vi "Destroy_ErrorHandler.vi"(8 "error in (no error)":errorcluster, 11 "ErrorHandler in":refnum<class "ErrorHandler.lvclass">) -> (0 "error out":errorcluster, 3 "ErrorHandler out":refnum<class "ErrorHandler.lvclass">)   [LabVIEW 2017, in "ErrorHandler.lvclass"]
doc: "Developed by Kevin Thompson\nkevin@thompsonengineering.net\n\nCopyright 2018\nThompson Engineering, LLC"
uses:
  ErrorHandler.lvclass
  TypeDef/TD GetSet ActionSelect--enum.ctl
  ErrorHandler.lvclass/ErrorHandler.ctl
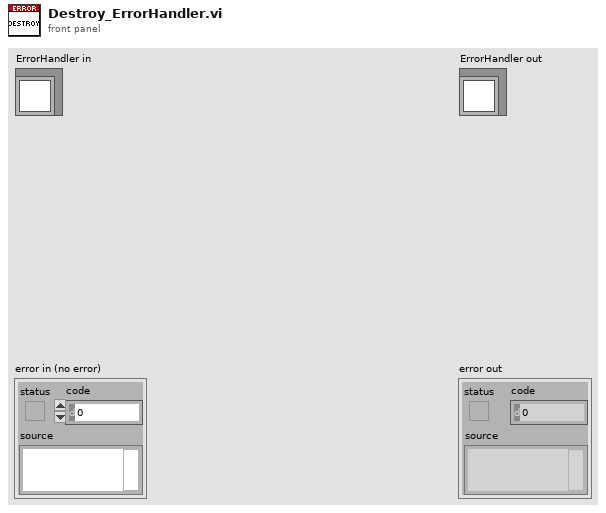
[diagram p1: front panel]
types:
  T1 = typedef "ErrorHandler.lvclass/TD GetSet ActionSelect--enum.ctl" = enum16{"Init", "Get", "Set"}
  T2 = typedef "ErrorHandler.lvclass/Public Events.ctl" = cluster{"ErrorRemote Ev":refnum<user-event>}
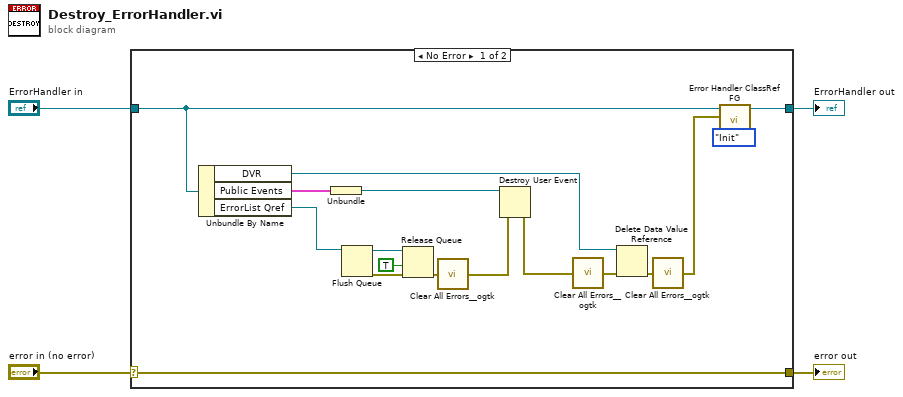
[diagram p0: block diagram]
diagram:
  n1 = case shown="No Error" "error in (no error)" {
    selector: "error in (no error)" -> [w21 w23]
    tunnel: [w21 w23] -> w3
    tunnel: [w7 w22] -> w1
    tunnel: "ErrorHandler in" -> [w8 w22]
    frame No Error {
      n2 = Unbundle By Name(w8) -> ("DVR"=w14:refnum<data-value>, "Public Events"=w16:T2, "ErrorList Qref"=w18:refnum<queue>)
      n3 = Unbundle(w16) -> ("ErrorRemote Ev"=w15:refnum<user-event>)
      n4 = Flush Queue(queue=w18) -> (queue out=w20:refnum<queue>, error out=w19:errorcluster)  [unwired: 1 in, 1 out]
      n5 = Release Queue(queue=w20, force destroy? (F)=TRUE, error in (no error)=w19) -> (error out=w13:errorcluster)  [unwired: 2 out]
      n6 = call <userlib>:"Clear All Errors__ogtk.vi"("Error In"=w13) -> ("Error Out"=w12:errorcluster)  [unwired: 3 in]
      n7 = Destroy User Event(user event=w15, error in=w12) -> (error out=w11:errorcluster)
      n8 = call <userlib>:"Clear All Errors__ogtk.vi"("Error In"=w11) -> ("Error Out"=w10:errorcluster)  [unwired: 3 in]
      n9 = Delete Data Value Reference(data value reference=w14, error in=w10) -> (error out=w6:errorcluster)  [unwired: 1 out]
      n10 = call <userlib>:"Clear All Errors__ogtk.vi"("Error In"=w6) -> ("Error Out"=w5:errorcluster)  [unwired: 3 in]
      n11 = call "Error Handler ClassRef FG.vi"("action (Get)"=TD_GetSet_ActionSelect--enum."Init", "error in (no error)"=w5, "ErrorHandler in"=w8) -> ("ErrorHandler out"=w7:refnum<class "ErrorHandler.lvclass">)  [unwired: 7 in, 1 out]
    }
    frame Error {
    }
  }
  "error out" <- w3
  "ErrorHandler out" <- w1
